vi "Get Most Recent Frame (if active).vi"(8 "error in (no error)":errorcluster, 11 "Orca-Flash 4.0 V2 in":refnum<class "Hamamatsu Camera.lvclass">) -> (0 "error out":errorcluster, 3 "Orca-Flash 4.0 V2 out":refnum<class "Hamamatsu Camera.lvclass">)   [LabVIEW 2023, in "Hamamatsu Camera.lvlib" / "Hamamatsu Camera.lvclass"]
uses:
  Hamamatsu Camera.lvclass
  C:/FlashGordon/Development/Hardware/Camera/Camera.lvclass
  C:/Program Files/National Instruments/LabVIEW 2023/vi.lib/ActorFramework/Actor/Actor.lvclass
  <vilib>/ActorFramework/Actor/Actor.lvclass/Actor.ctl
  Application Messages/New Frame Notify Msg/New Frame Notify Msg.lvclass/New Frame Notify Msg.ctl
  <vilib>/ActorFramework/Message Enqueuer/Message Enqueuer.lvclass/Message Enqueuer.ctl
  <vilib>/ActorFramework/Message Enqueuer/Enqueue.vi
  Application Messages/New Frame Notify Msg/New Frame Notify Msg.lvclass
  C:/Program Files/National Instruments/LabVIEW 2023/vi.lib/ActorFramework/Message/Message.lvclass
  Resources/GLOBAL/GLOBAL Time-critical.vi
  <vilib>/ActorFramework/Message Priority Queue/Priority Enqueue.vi
  Hamamatsu Camera.lvclass/Hamamatsu Camera.ctl
  Camera/Camera.lvlib
  <vilib>/ActorFramework/Actor/Actor.lvclass
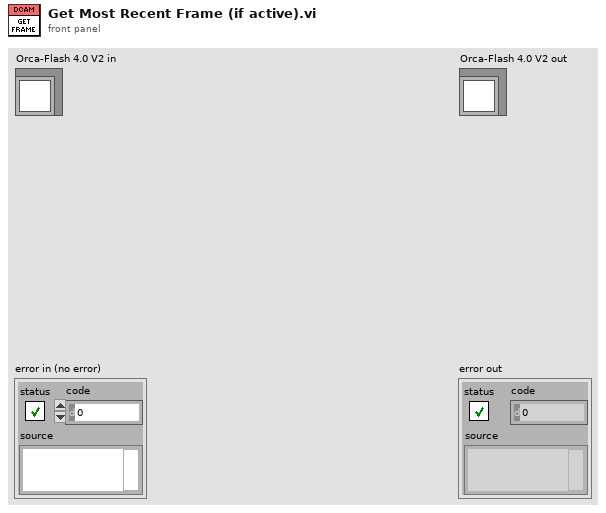
[diagram p1: front panel]
types:
  T1 = typedef "Physical Camera Assignment.ctl" = cluster{"Channel Name":string, "Serial Number":string, "Flip Vertically":bool, "Flip Horizontally":bool, "wavelength":i16, "photonsPerCount":dbl[]}
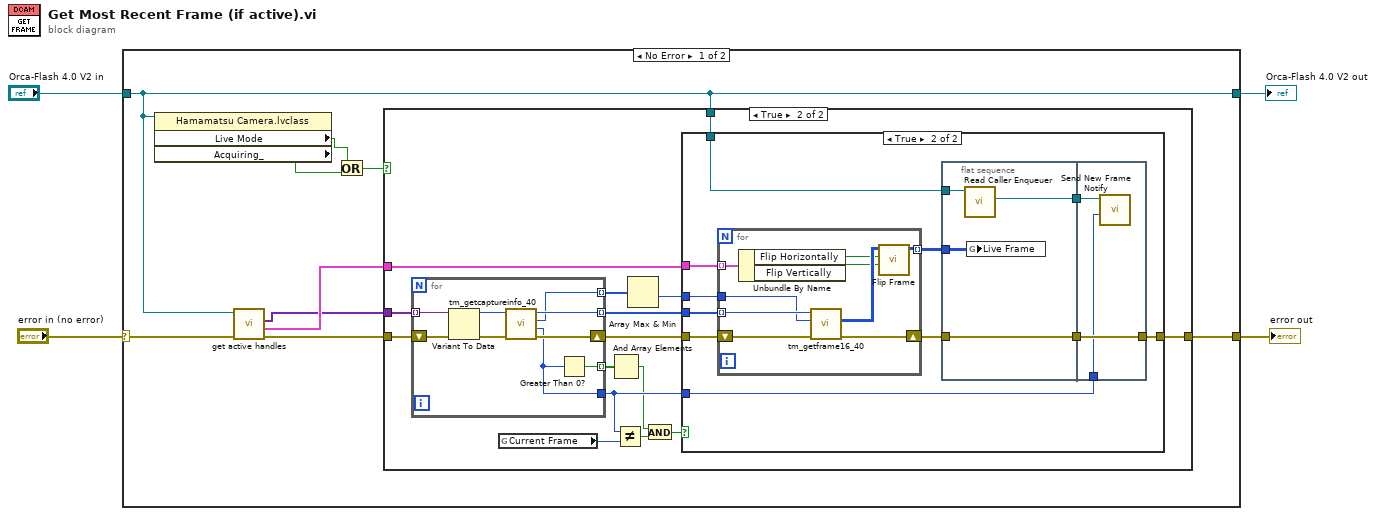
[diagram p0: block diagram]
diagram:
  n1 = case shown="No Error" "error in (no error)" {
    selector: "error in (no error)" -> [w8 w68]
    tunnel: [w12 w68] -> w1
    tunnel: [w9 w67] -> w2
    tunnel: "Orca-Flash 4.0 V2 in" -> [w9 w67]
    frame No Error {
      n2 = property class="Hamamatsu Camera.lvclass"(reference=w9) -> ("Live Mode"=w13:bool, "Acquiring_"=w10:bool)  [unwired: 1 in, 2 out]
      n3 = call-dynamic "get active handles.vi"("error in (no error)"=w8, "Camera in"=w9) -> ("error out"=w7:errorcluster, "Active Cameras"=w6:T1[], "Handles"=w5:variant[])  [unwired: 5 in, 2 out]
      n4 = Or(x=w13, y=w10) -> (x .or. y?=w11:bool)
      n5 = case shown="True" w11 {
        tunnel: w7 -> [w14 w26]
        tunnel: [w14 w29] -> w12
        tunnel: w6 -> [_ w24]
        tunnel: w5 -> [_ w23]
        tunnel: w9 -> [_ w17]
        frame False {
        }
        frame True {
          n6 = for {
            tunnel: w23 -> [w30] mode=indexing
            tunnel: [w38] -> w28 mode=indexing
            tunnel: [w36] -> w16 mode=indexing
            tunnel: [w35] -> w21
            shift-right: [w37] -> w27
            shift-left: w26 -> [w33]
            tunnel: [w34] -> w25 mode=indexing
            n7 = Variant To Data(error in=w33, Variant=w30) -> (data=w31:u32, error out=w32:errorcluster)  [unwired: 1 in]
            n8 = call <userlib>:"tm_getcaptureinfo_40.vi"("error in (no error)"=w32, "Handle in"=w31) -> ("error out"=w37:errorcluster, "Frame Count"=w35:i32, "Frame Index"=w36:i32, "Handle out"=w38:u32)  [unwired: 6 in]
            n9 = Greater Than 0?(x=w35) -> (x > 0?=w34:bool)
          }
          n10 = global read "GLOBAL Time-critical.vi" "Current Frame"() -> (w22:i32)
          n11 = And Array Elements(Boolean array=w25) -> (logical AND=w19:bool)
          n12 = Not Equal?(x=w21, y=w22) -> (x != y?=w20:bool)
          n13 = Array Max & Min(array=w16) -> (min value=w15:i32)  [unwired: 3 out]
          n14 = And(x=w19, y=w20) -> (x .and. y?=w18:bool)
          n15 = case shown="True" w18 {
            tunnel: [w39 w45] -> w29
            tunnel: w24 -> [_ w50]
            tunnel: w28 -> [_ w48]
            tunnel: w27 -> [w39 w47]
            tunnel: w21 -> [_ w42]
            tunnel: w17 -> [_ w44]
            tunnel: w15 -> [_ w40]
            frame False {
            }
            frame True {
              n16 = for {
                tunnel: w48 -> [w63] mode=indexing
                shift-right: [w66] -> w46
                shift-left: w47 -> [w64]
                tunnel: w50 -> [w65] mode=indexing
                tunnel: [w62] -> w49 mode=indexing
                tunnel: w40 -> [w58]
                n17 = Unbundle By Name(w65) -> ("Flip Horizontally"=w60:bool, "Flip Vertically"=w59:bool)
                n18 = call <userlib>:"tm_getframe16_40.vi"("error in (no error)"=w64, "Frame Index"=w58, "Handle in"=w63) -> ("error out"=w66:errorcluster, "Data"=w61:u16[][])  [unwired: 5 in, 2 out]
                n19 = call "Flip Frame.vi"("Flip Vertically"=w59, "Flip Horizontally"=w60, "Input Array"=w61) -> ("output array"=w62:u16[][])  [unwired: 8 in]
              }
              n20 = flat-sequence {
                tunnel: w49 -> [w54]
                tunnel: w46 -> [w53]
                tunnel: w44 -> [w52]
                tunnel: [w53] -> w43
                tunnel: [w51] -> w41
                tunnel: [w57] -> w45
                tunnel: w43 -> [w57]
                tunnel: w42 -> [w56]
                tunnel: w41 -> [w55]
                frame #0 {
                  n21 = call <vilib>:"Read Caller Enqueuer.vi"("Actor"=w52) -> ("Caller Enqueuer"=w51:refnum<class "Message Enqueuer.lvclass">)  [unwired: 10 in]
                  n22 = global write "GLOBAL Time-critical.vi" "Live Frame"(w54) -> ()
                }
                frame #1 {
                  n23 = call "Send New Frame Notify.vi"("Frame Number\n(starts with 1)"=w56, "Message Enqueuer"=w55) -> ()  [unwired: 8 in, 2 out]
                }
              }
            }
          }
        }
      }
    }
    frame Error {
    }
  }
  "error out" <- w1
  "Orca-Flash 4.0 V2 out" <- w2
